vi "generate_config.vi"(0 "new task name":string, 1 "Generate config":T1={"maximum value"=5.0, "minimum value"=-5.0, "phase"=180.0, "amplitude"=1.0, "frequency"=10.0, "Wave Type"=0, "offset"=0.0} {"offset" format="%0.2p"; "Wave Type" items=["Sine", "Square", "Triangle", "Sawtooth", "DC Signal"]; "frequency" format="%0.2p"; "amplitude" format="%0.2p"}, 2 "Analog Out Channels":cluster{"0":bool, "1":bool}={"0"=TRUE, "1"=FALSE}) -> (3 "task out":refnum<k21>, 4 "signal Generated":waveform(dbl)(graph), 5 "real frequency(Hz)":dbl, 6 "error out":errorcluster)   [LabVIEW 2017]
uses:
  <vilib>/DAQmx/write.llb/DAQmx Write (Analog Wfm 1Chan NSamp).vi
  <vilib>/DAQmx/create/channels.llb/DAQmx Create Channel (AO-Voltage-Basic).vi
  <vilib>/DAQmx/configure/timing.llb/DAQmx Timing (Use Waveform).vi
  <vilib>/DAQmx/miscellaneous.llb/DAQmx Fill In Error Info.vi
  <instrlib>/NI USB-6356/NI USB-6356.lvlib
panel:
  in  "error in":errorcluster
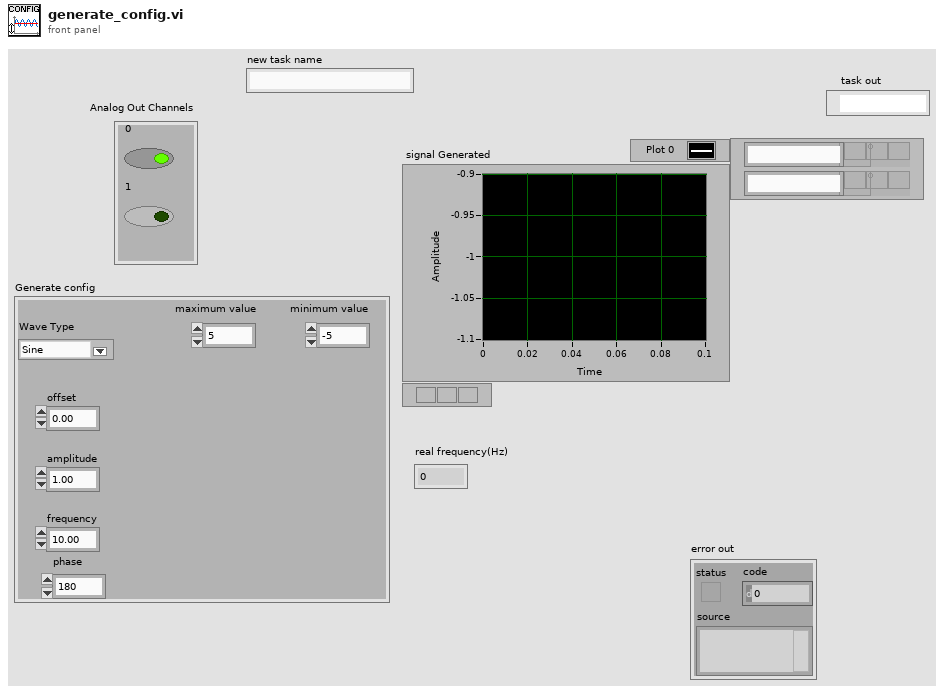
[diagram p1: front panel]
types:
  T1 = cluster{"maximum value":dbl, "minimum value":dbl, "phase":dbl, "amplitude":dbl, "frequency":dbl, "Wave Type":u16, "offset":dbl}
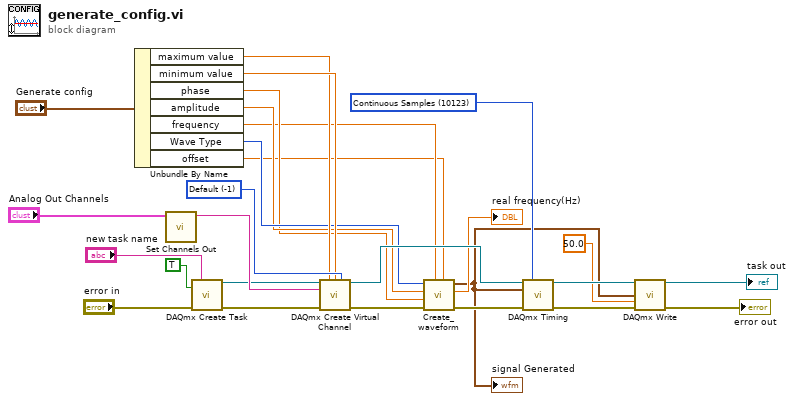
[diagram p0: block diagram]
diagram:
  w21 = 10123 items=["Finite Samples"=10178, "Continuous Samples"=10123, "Hardware Timed Single Point"=12522] ("sample mode")
  w27 = -1 items=["Default"=-1, "RSE"=10083, "Differential"=10106, "Pseudodifferential"=12529] ("output terminal configuration")
  n1 = Unbundle By Name("Generate config") -> ("maximum value"=w7:dbl, "minimum value"=w8:dbl, "phase"=w4:dbl, "amplitude"=w5:dbl, "frequency"=w3:dbl, "Wave Type"=w6:u16, "offset"=w2:dbl)
  n2 = call <instrlib>:"Set Channels Out.vi"("Analog Out Channels"="Analog Out Channels") -> ("String"=w26:string)  [unwired: 10 in]
  n3 = call <vilib>:"DAQmx Create Task.vi"("new task name"="new task name", "auto cleanup"=TRUE, "error in"="error in") -> ("task out"=w14:refnum<k21>, "error out"=w13:errorcluster)  [unwired: 11 in]
  n4 = call-poly <vilib>:"DAQmx Create Virtual Channel.vi"("task in"=w14, "maximum value"=w7, "minimum value"=w8, "output terminal configuration"=w27, "physical channels"=w26, "error in"=w13) -> ("task out"=w25:refnum<k21>, "error out"=w24:errorcluster)  [unwired: 8 in]
  n5 = call "Create_waveform.vi"("offset"=w2, "frequency"=w3, "error in"=w24, "phase"=w4, "amplitude"=w5, "Wave Type"=w6) -> ("error out"=w17:errorcluster, "real frequency(Hz)"=→"real frequency(Hz)":dbl, "signal Generated"=w10:waveform(dbl))  [unwired: 3 in]
  "signal Generated" <- w10
  n6 = call-poly <vilib>:"DAQmx Timing.vi"("task/channels in"=w25, "sample mode"=w21, "waveform"=w10, "error in"=w17) -> ("task out"=w22:refnum<k21>, "error out"=w23:errorcluster)  [unwired: 10 in]
  n7 = call-poly <vilib>:"DAQmx Write.vi"("task/channels in"=w22, "data"=w10, "timeout"=50.0, "error in"=w23) -> ("task out"=→"task out":refnum<k21>, "error out"=→"error out":errorcluster)  [unwired: 9 in, 1 out]
